vi "Radar Plot - Sinan.vi"() -> ()   [LabVIEW 2017]
uses:
  <vilib>/picture/picture.llb/imagedata.ctl
panel:
  in  "Visible Section":u16(ring)=8
  in  "Target":cluster{"r":i16, "theta":i16}={"r"=0, "theta"=57} {"theta" min=-90 max=90 step=5; "r" min=0 max=100 step=10}
  in  "stop":bool
  out "2D Picture":picture
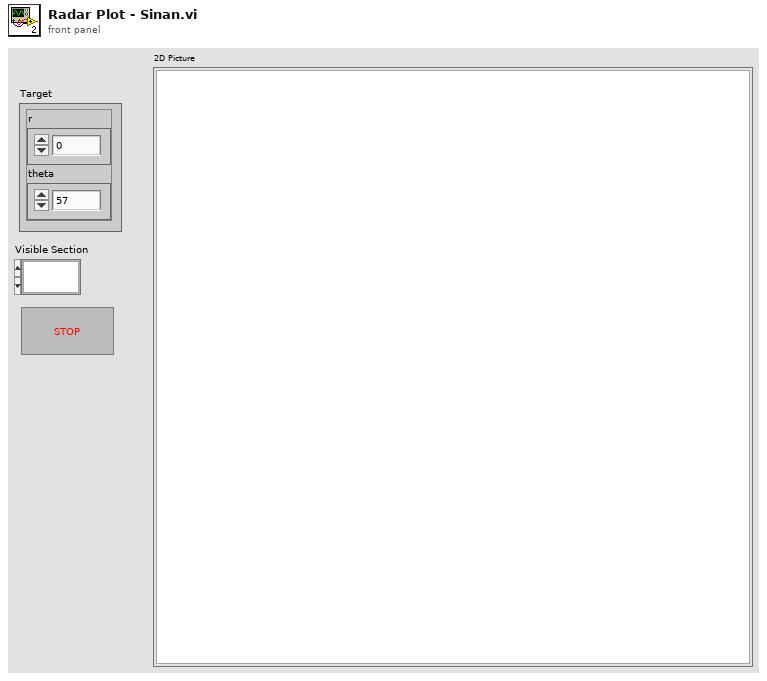
[diagram p1: front panel]
types:
  T1 = typedef "imagedata.ctl" = cluster{"image type":i32, "image depth":i32, "image":u8[], "mask":u8[], "colors":u32[], "Rectangle":cluster{"left":i16, "top":i16, "right":i16, "bottom":i16}}
  T2 = cluster{"maximum":dbl, "minimum":dbl, "clip to min":bool, "log?(F)":bool, "grid color":u32, "plot color":u32, "format and precision":cluster{"format":enum8{"Decimal", "Scientific", "Engineering", "Binary", "Octal", "Hex"}, "precision":u8}, "visible section":u16}
  T3 = cluster{"pixel center":cluster{"x":i16, "y":i16}, "scale factors":cluster{"a":dbl, "b":dbl, "log?":bool}, "grid color":u32, "start angle":dbl, "end angle":dbl, "tick length":i16, "pixel radius":i32}
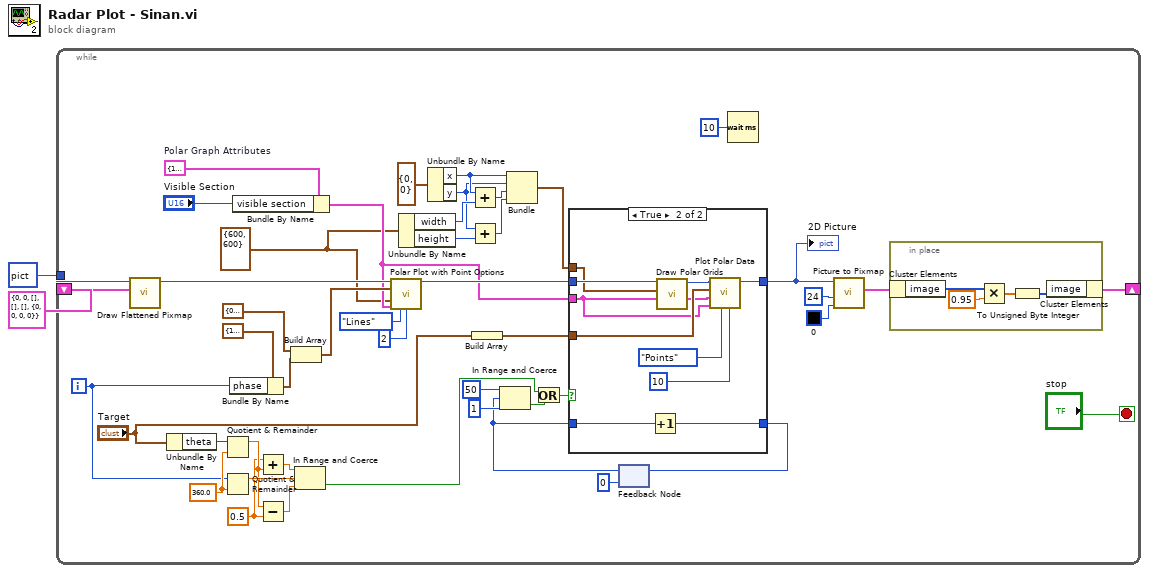
[diagram p0: block diagram]
diagram:
  n1 = while {
    shift-right: [w47] -> _
    shift-left: T1 {"image type"=0, "image depth"=0, "image"=[], "mask"=[], "colors"=[], "Rectangle"={"left"=0, "top"=0, "right"=0, "bottom"=0}} ("image data") -> [w46]
    tunnel: picture data[5B] ("2D Picture") -> [w45]
    i -> [w15]
    stop <- "stop" stop-if-true
    w3 = cluster{"width":i16, "height":i16} {"width"=600, "height"=600} ("dimensions (w,h)")
    w16 = 0.5
    w20 = 360.0 ("y")
    w36 = T2 {"maximum"=100.0, "minimum"=2.0, "clip to min"=TRUE, "log?(F)"=FALSE, "grid color"=9868950, "plot color"=65280, "format and precision"={"format"=enum."Decimal", "precision"=1}, "visible section"=0}  # Polar Graph Attributes
    n2 = call <vilib>:"Draw Flattened Pixmap.vi"("image data"=w46, "picture"=w45) -> ("new picture"=w37:picture)  [unwired: 7 in]
    n3 = Unbundle By Name("Target") -> ("theta"=w13:i16)
    n4 = Quotient & Remainder(x=w13, y=w20) -> (x-y*floor(x/y)=w19:dbl)  [unwired: 1 out]
    n5 = Quotient & Remainder(x=w15, y=w20) -> (x-y*floor(x/y)=w21:dbl)  [unwired: 1 out]
    n6 = Bundle By Name(cluster=cluster{"magnitude":dbl, "phase":dbl} {"magnitude"=100.0, "phase"=0.0}, "phase"=w15) -> (w44:cluster{"magnitude":dbl, "phase":dbl})
    n7 = Bundle By Name(cluster=w36, "visible section"="Visible Section") -> (w22:T2)
    n8 = Add(x=w16, y=w19) -> (x+y=w17:dbl)
    n9 = Subtract(x=w19, y=w16) -> (x-y=w18:dbl)
    n10 = Build Array(cluster{"magnitude":dbl, "phase":dbl} {"magnitude"=0.0, "phase"=0.0}, w44) -> (w40:cluster{"magnitude":dbl, "phase":dbl}[])
    n11 = In Range and Coerce(upper limit=w17, x=w21, lower limit=w18) -> (In Range?=w9:bool)  [unwired: 1 out]
    n12 = call <vilib>:"Polar Plot with Point Options.vi"("picture"=w37, "data array [mag, phase (deg)]"=w40, "dimensions (w,h)"=w3, "polar attributes"=w22, "Lines/Points"=enum16{"Lines", "Points"}."Lines", "Size"=u16 2) -> ("new picture"=w33:picture)  [unwired: 9 in]
    n13 = Unbundle By Name(w3) -> ("width"=w32:i16, "height"=w31:i16)
    n14 = Unbundle By Name(cluster{"x":i16, "y":i16} {"x"=0, "y"=0} ("input cluster")) -> ("x"=w30:i16, "y"=w29:i16)
    n15 = Add(x=w30, y=w32) -> (x+y=w28:i16)
    n16 = Add(x=w29, y=w31) -> (x+y=w27:i16)
    n17 = Build Array("Target") -> (w24:cluster{"r":i16, "theta":i16}[])
    n18 = Bundle("x"=w30, "y"=w29, w28, w27) -> (w25:cluster{"x":i16, "y":i16, i16, i16})  [unwired: 1 in]
    n19 = feedback #1(u16 0) -> (w5:u16)
    n20 = In Range and Coerce(upper limit=u16 50 ("y"), x=w5, lower limit=u16 1) -> (In Range?=w11:bool)  [unwired: 1 out]
    n21 = Or(x=w9, y=w11) -> (x .or. y?=w10:bool)
    n22 = case shown="True" w10 {
      tunnel: [w50 w61] -> w34
      tunnel: w33 -> [w50 w60]
      tunnel: w25 -> [_ w59]
      tunnel: w24 -> [_ w58]
      tunnel: w22 -> [_ w57]
      tunnel: w5 -> [_ w52]
      tunnel: [_ w51] -> w7
      frame False {
      }
      frame True {
        n23 = Increment(x=w52) -> (x+1=w51:u16)
        n24 = call <vilib>:"Draw Polar Grids.vi"("polar attributes"=w57, "rect"=w59, "picture"=w60) -> ("grid measurements"=w53:T3, "new picture"=w56:picture)  [unwired: 7 in]
        n25 = call <vilib>:"Plot Polar Data.vi"("Size"=u16 10, "Lines/Points"=enum16{"Lines", "Points"}."Points", "polar attributes"=w57, "grid measurements"=w53, "polar data"=w58, "picture"=w56) -> ("new picture"=w61:picture)  [unwired: 3 in]
      }
    }
    "2D Picture" <- w34
    n26 = feedback-in #1(w7) -> ()
    n27 = Wait (ms)(milliseconds to wait=u32 10) -> ()  [unwired: 1 out]
    n28 = call <vilib>:"Picture to Pixmap.vi"("Background Color"=u32 0, "depth"=24, "picture"=w34) -> ("image data"=w48:T1)  [unwired: 7 in, 1 out]
    n29 = in-place {
      n30 = in-place-cluster #2(w48) -> ("image"=w65:u8[])
      n31 = Multiply(x=w65, y=0.95) -> (x*y=w63:dbl[])
      n32 = To Unsigned Byte Integer(number=w63) -> (unsigned 8bit integer=w62:u8[])
      n33 = in-place-cluster #2("image"=w62) -> (w47:T1)
    }
  }
